vi "Vision Process.vi"(11 "Vision String":string) -> (3 "Default Values":dbl[](array[numeric]))   [LabVIEW 2018]
uses:
  TypeDefs/Teleop Data Cluster.ctl
  TypeDefs/Joystick Buttons.ctl
panel:
  in  "Teleop Data Cluster":T1
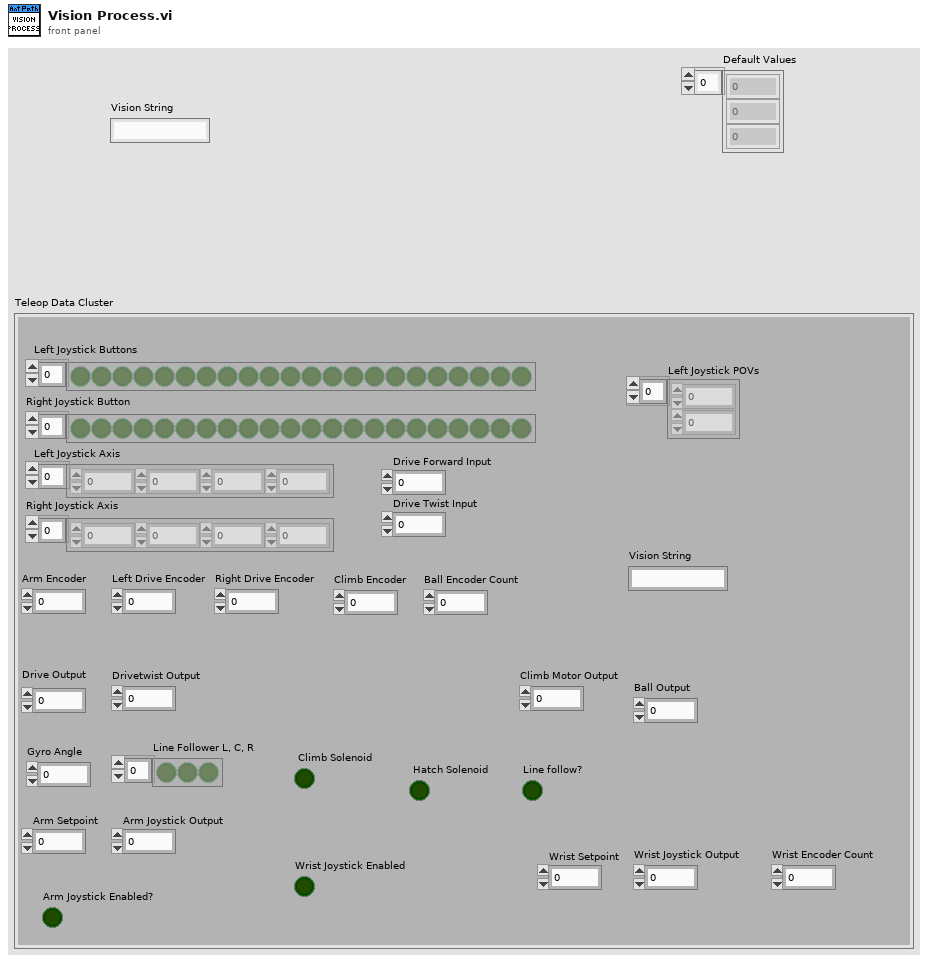
[diagram p1: front panel]
types:
  T1 = typedef "Teleop Data Cluster.ctl" = cluster{"Drive Forward Input ":dbl, "Drive Twist Input":dbl, "Drive Output":dbl, "Drivetwist Output":dbl, "Left Joystick Buttons":bool[], "Left Joystick Axis":dbl[], "Right Joystick Axis":dbl[], "Right Joystick Button":bool[], "Arm Encoder":dbl, "Left Drive Encoder":dbl, "Right Drive Encoder":dbl, "Gyro Angle ":dbl, "Arm Joystick Output  ":dbl, "Line Follower L, C, R ":bool[], "Line follow?":bool, " Climb Solenoid":bool, "Wrist Encoder Count":dbl, "Wrist Joystick Output":dbl, "Ball Encoder Count":dbl, "Ball Output":dbl, "Climb Encoder":dbl, "Climb Motor Output":dbl, " Hatch Solenoid":bool, "Arm Setpoint ":dbl, "Wrist Setpoint ":dbl, "Arm Joystick Enabled?":bool, "Wrist Joystick Enabled":bool, "Vision String":string, "Left Joystick POVs":i16[]}
  T2 = typedef "Joystick Buttons.ctl" = enum16{"Trigger", "Thumb", "Top 3", "Top 4", "Top 5", "Top 6", "Bottom 7", "Bottom 8", "Bottom 9", "Bottom 10", "Bottom 11", "Bottom 12"}
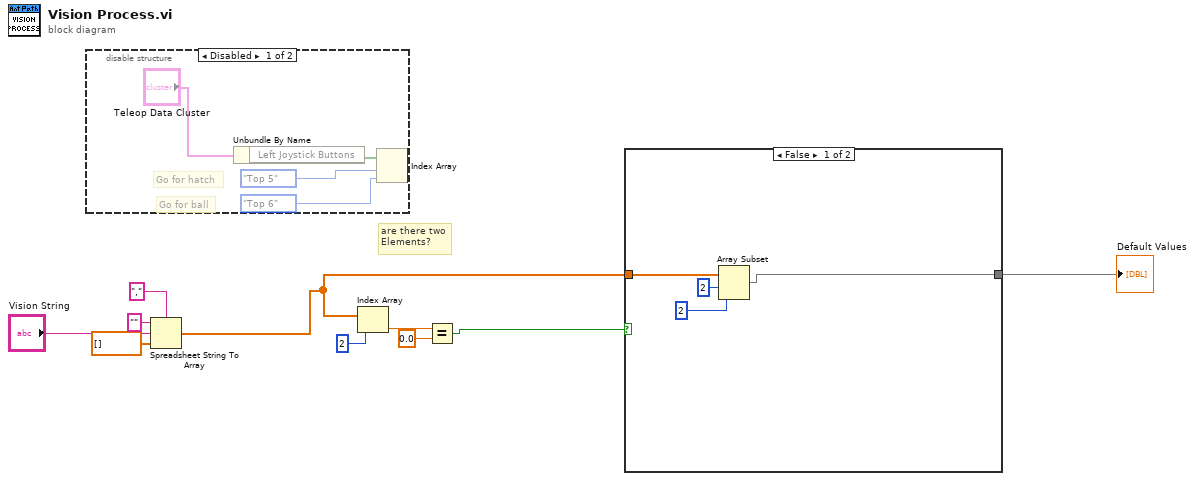
[diagram p0: block diagram]
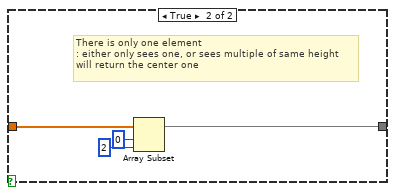
[diagram p3: hidden frame]
diagram:
  # "are there two\nElements?"
  n1 = disable-structure shown="Disabled" {
    frame Disabled {
      # "Go for ball"
      # "Go for hatch"
      n2 = Unbundle By Name("Teleop Data Cluster") -> ("Left Joystick Buttons"=w13:bool[])
      n3 = Index Array(array=w13, index #1=Joystick_Buttons."Top 5" ("Enum"), index #2=Joystick_Buttons."Top 6" ("Enum")) -> ()  [unwired: 2 out]
    }
    frame Enabled {
    }
  }
  n4 = Spreadsheet String To Array(delimiter (Tab)=",", format string="", spreadsheet string="Vision String", array type (2D Dbl)=dbl[] []) -> (array=w1:dbl[])
  n5 = Index Array(array=w1, index=2) -> (element=w9:dbl)
  n6 = Equal?(x=w9, y=0.0) -> (x = y?=w6:bool)
  n7 = case shown="False" w6 {
    tunnel: w1 -> [w18 w22]
    tunnel: [w15 w21] -> w7
    frame False {
      n8 = Array Subset(array=w18, index=2, length=2) -> (w15:dbl[])
    }
    frame True {
      # "There is only one element\n: either only sees one, or sees multiple of same height\nwill return the center one"
      n9 = Array Subset(array=w22, index=0, length=2) -> (w21:dbl[])
    }
  }
  "Default Values" <- w7
